vi "LoadModel.vi"(8 "error in (no error)":errorcluster, 11 "View in":refnum<class "View.lvclass">) -> (0 "error out":errorcluster, 3 "View out":refnum<class "View.lvclass">)   [LabVIEW 2020, in "Page1.lvlib" / "View.lvclass"]
uses:
  View.lvclass
  View.lvclass/View.ctl
  Controller/Controller.lvclass
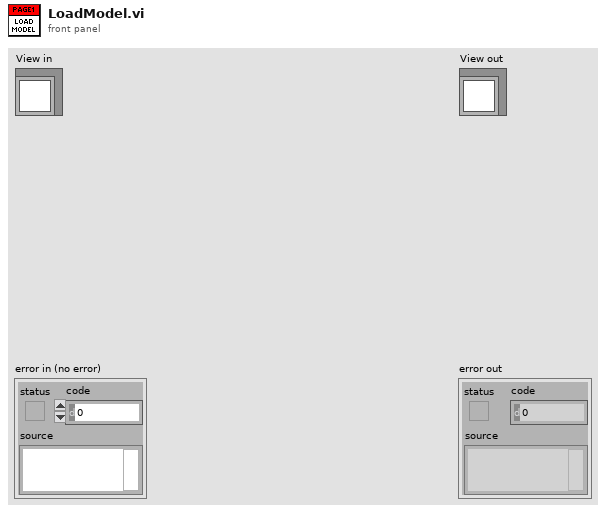
[diagram p1: front panel]
types:
  T1 = cluster{"Main Test Folder":refnum<vi>, "Time (s)":refnum<vi>, "Setting":refnum<vi>}
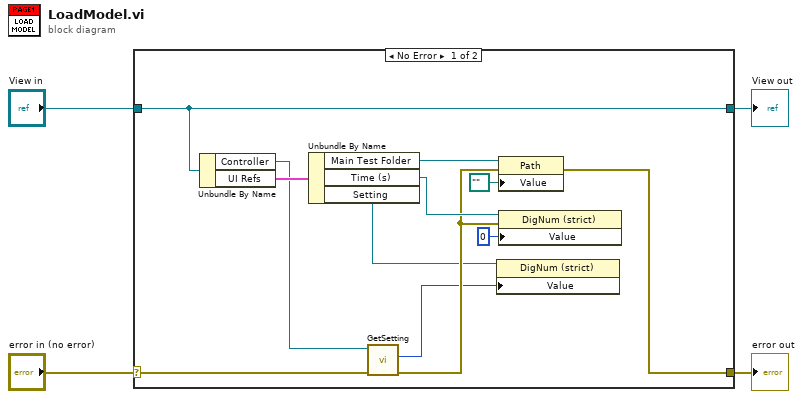
[diagram p0: block diagram]
diagram:
  n1 = case shown="No Error" "error in (no error)" {
    selector: "error in (no error)" -> [w6 w18]
    tunnel: [w11 w18] -> w3
    tunnel: [w14 w17] -> w1
    tunnel: "View in" -> [w14 w17]
    frame No Error {
      n2 = Unbundle By Name(w14) -> ("Controller"=w7:refnum<class "Controller.lvclass">, "UI Refs"=w16:T1)
      n3 = Unbundle By Name(w16) -> ("Main Test Folder"=w15:refnum<vi>, "Time (s)"=w13:refnum<vi>, "Setting"=w9:refnum<vi>)
      n4 = call "GetSetting.vi"("error in (no error)"=w6, "Controller in"=w7) -> ("error out"=w10:errorcluster, "Setting"=w8:u32)  [unwired: 7 in, 1 out]
      n5 = property class="DigNum (strict)"(reference=w9, "Value"=w8) -> ()  [unwired: 1 in, 2 out]
      n6 = property class="Path"(reference=w15, error in=w10, "Value"=path "") -> (error out=w11:errorcluster)  [unwired: 1 out]
      n7 = property class="DigNum (strict)"(reference=w13, error in=w10, "Value"=u32 0) -> ()  [unwired: 2 out]
    }
    frame Error {
    }
  }
  "error out" <- w3
  "View out" <- w1
